vi "compact form to sym matrix.vi"(10 "Compact Form":dbl[](array[numeric]), 11 "Preallocated Matrix":T1) -> (3 "Symmetric Matrix":T1)   [LabVIEW 2018, in "NI_AALPro.lvlib"]
uses:
  <vilib>/Analysis/NI_AALPro.lvlib
  RealMatrix.ctl
  <resource>/lvanlys.dll
  NI_Matrix.lvlib
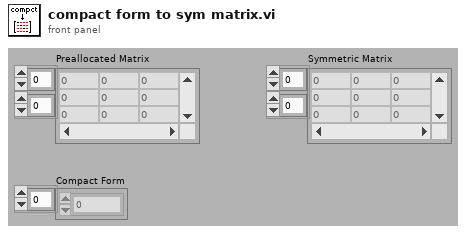
[diagram p1: front panel]
types:
  T1 = typedef "NI_Matrix.lvlib/RealMatrix.ctl" = dbl[][]
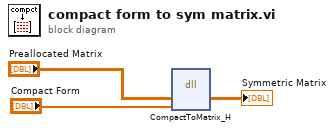
[diagram p0: block diagram]
diagram:
  n1 = dll-call lib="C:/Program Files (x86)/National Instruments/LabVIEW 2018/resource/lvanlys.*" fn="CompactToMatrix_H"("matrixH"="Preallocated Matrix", "aH"="Compact Form") -> ("matrixH"=→"Symmetric Matrix":dbl[][])  [unwired: 5 in, 2 out]
